vi "雨流计数法.vi"(2 "Data":i32[](array[numeric]), 3 "数据个数":i32=20) -> (0 "Cluster 2":T1, 1 "Cluster":T2)   [LabVIEW 2019]
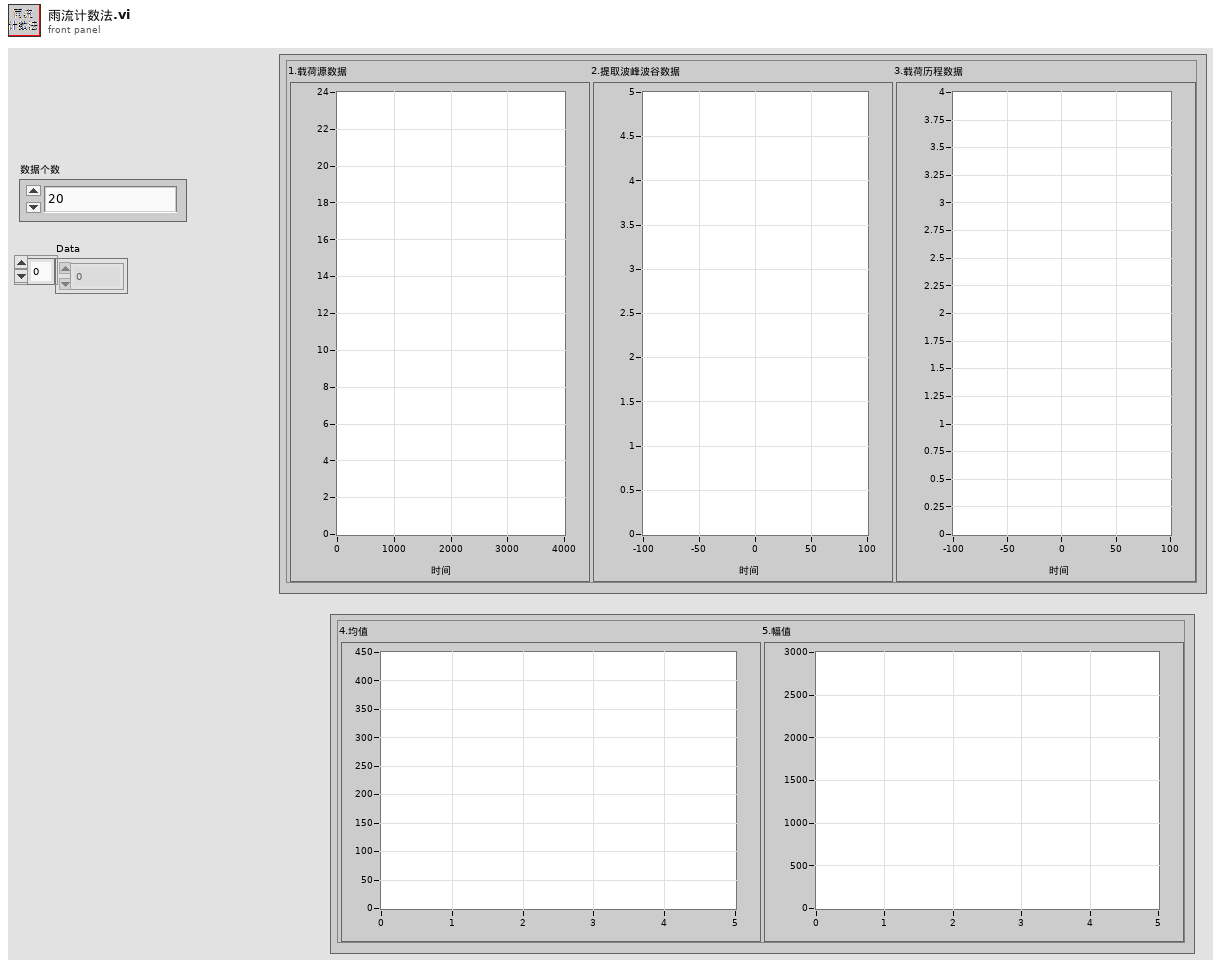
[diagram p1: front panel]
types:
  T1 = cluster{"4.均值":cluster{"子数组2":i32[], "子数组1":dbl[]}, "5.幅值":cluster{"子数组2":i32[], "子数组1":dbl[]}}
  T2 = cluster{"1.载荷源数据":cluster{"Data":i32[], "label":i32[]}, "2.提取波峰波谷数据":cluster{"时间戳":i32[], "峰谷戳":i32[]}, "3.载荷历程数据":cluster{"子数组1":i32[], "子数组2":i32[]}}
  T3 = cluster{cluster{"Data":i32[], "label":i32[]}, cluster{"子数组1":i32[], "子数组2":i32[]}, cluster{"子数组1":i32[], "子数组2":i32[]}}
  T4 = cluster{cluster{"子数组2":i32[], "子数组1":dbl[]}, cluster{"子数组2":i32[], "子数组1":dbl[]}}
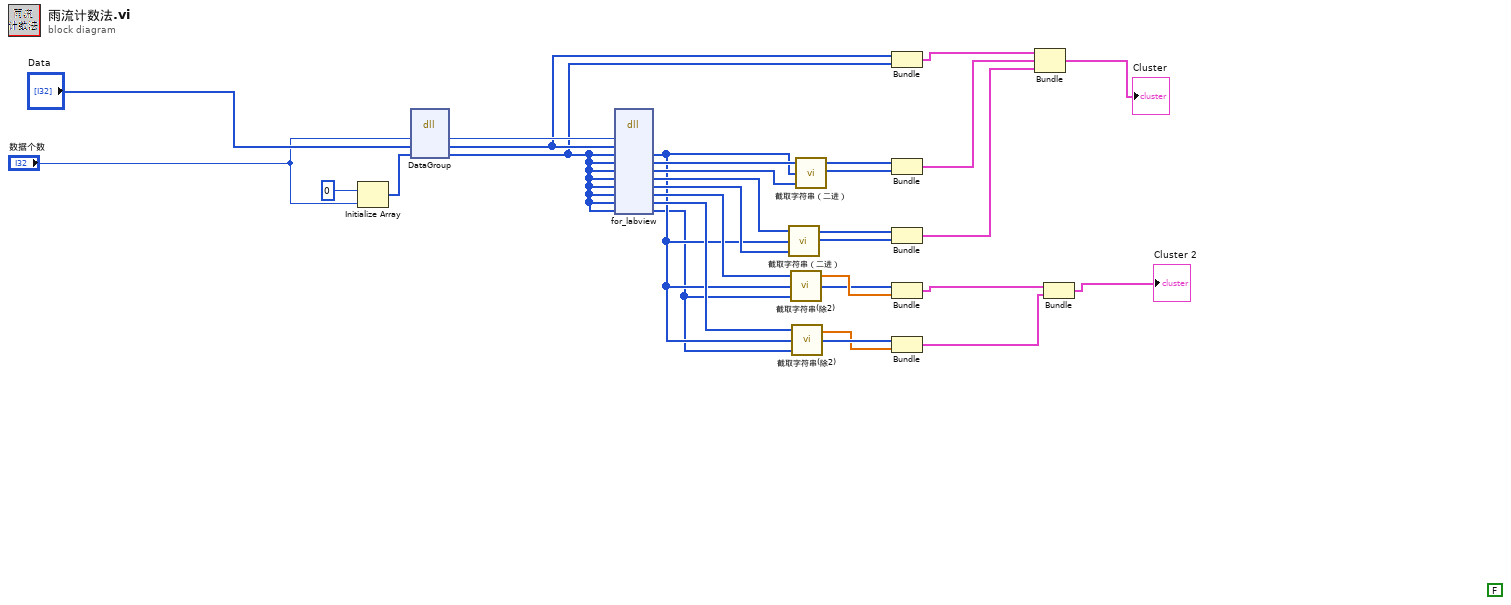
[diagram p0: block diagram]
diagram:
  (unwired) FALSE
  n1 = Initialize Array(0 ("元素"), "数据个数") -> (w28:i32[])
  n2 = dll-call lib="PTH2oabs E\nLabVIEW工程上位机设计2020.2.4雨流计数法雨流计数法x64Debug数据成组.dll" fn="DataGroup"("Num"="数据个数", "Data"="Data", "label"=w28) -> ("Num"=w29:i32, "Data"=w27:i32[], "label"=w14:i32[])  [unwired: 4 in, 2 out]
  n3 = dll-call lib="PTH2oabs E\nLabVIEW工程上位机设计2020.2.4雨流计数法雨流计数法x64Debug导出为DLL.dll" fn="for_labview"("长度"=w29, "源数据"=w27, "时间"=w14, "峰谷提取数组"=w14, "l1"=w14, "载荷历程调整数组"=w14, "l2"=w14, "均值"=w14, "幅值"=w14, "幅均长度"=w14) -> ("时间"=w16:i32[], "峰谷提取数组"=w22:i32[], "l1"=w21:i32[], "载荷历程调整数组"=w20:i32[], "l2"=w19:i32[], "均值"=w18:i32[], "幅值"=w17:i32[], "幅均长度"=w15:i32[])  [unwired: 6 in, 2 out]
  n4 = call "截取字符串（二进）.vi"("长度"=w19, "数组 2"=w16, "数组1"=w20) -> ("子数组2"=w25:i32[], "子数组1"=w24:i32[])  [unwired: 1 in]
  n5 = call "截取字符串(除2).vi"("长度"=w15, "数组 2"=w16, "数组1"=w18) -> ("子数组2"=w10:i32[], "子数组1"=w13:dbl[])  [unwired: 1 in]
  n6 = call "截取字符串(除2).vi"("长度"=w15, "数组 2"=w16, "数组1"=w17) -> ("子数组2"=w12:i32[], "子数组1"=w11:dbl[])  [unwired: 1 in]
  n7 = call "截取字符串（二进）.vi"("长度"=w21, "数组 2"=w16, "数组1"=w22) -> ("子数组2"=w26:i32[], "子数组1"=w23:i32[])  [unwired: 1 in]
  n8 = Bundle("Data"=w27, "label"=w14) -> (w9:cluster{"Data":i32[], "label":i32[]})  [unwired: 1 in]
  n9 = Bundle("子数组1"=w23, "子数组2"=w26) -> (w8:cluster{"子数组1":i32[], "子数组2":i32[]})  [unwired: 1 in]
  n10 = Bundle("子数组1"=w24, "子数组2"=w25) -> (w7:cluster{"子数组1":i32[], "子数组2":i32[]})  [unwired: 1 in]
  n11 = Bundle("子数组2"=w10, "子数组1"=w13) -> (w5:cluster{"子数组2":i32[], "子数组1":dbl[]})  [unwired: 1 in]
  n12 = Bundle("子数组2"=w12, "子数组1"=w11) -> (w4:cluster{"子数组2":i32[], "子数组1":dbl[]})  [unwired: 1 in]
  n13 = Bundle(w9, w8, w7) -> (→"Cluster":T3)  [unwired: 1 in]
  n14 = Bundle(w5, w4) -> (→"Cluster 2":T4)  [unwired: 1 in]
